vi "ComputeFourierPhaseOfPeakSF.vi"(6 "Header":T1, 9 "Search SF Limit":i32=20, 10 "FFT size":i32=256, 11 "Scan Frame":dbl[][](array[numeric])) -> (0 "Col Shift Element Number":i32, 1 "Vertical SF Phase":dbl, 2 "Row Shift Element Numbert":i32, 3 "Horizontal SF Phase":dbl)   [LabVIEW 2014]
uses:
  <vilib>/Analysis/baseanly.llb/Mean (DBL).vi
  <vilib>/Analysis/2dsp.llb/Real FFT.vi
  <vilib>/Analysis/NI_AALPro.lvlib
  <vilib>/Analysis/NI_AALBase.lvlib
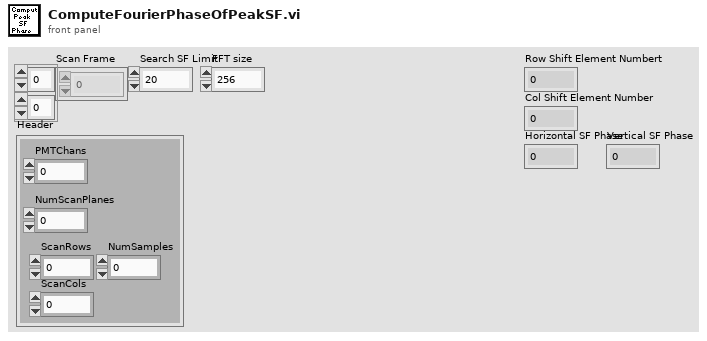
[diagram p1: front panel]
types:
  T1 = cluster{"PMTChans":i32, "NumScanPlanes":i32, "ScanRows":i32, "ScanCols":i32, "NumSamples":i32}
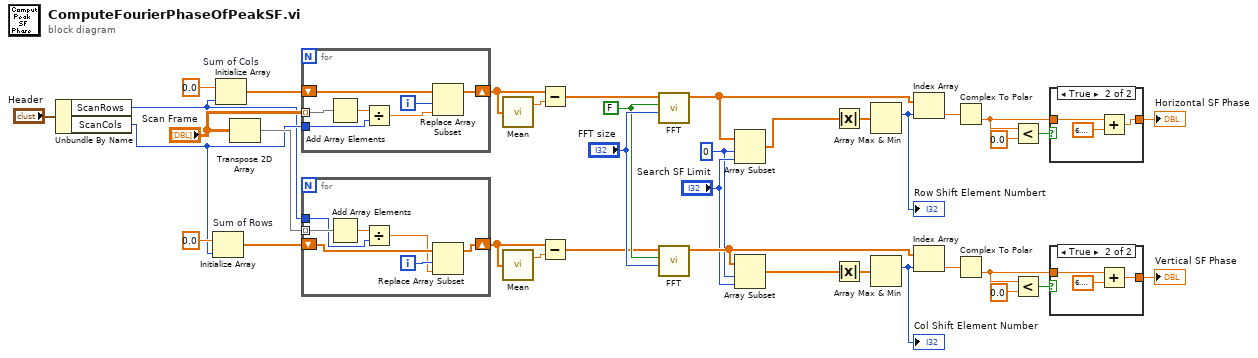
[diagram p0: block diagram]
diagram:
  w1 = 0 ("index")
  w29 = FALSE ("shift?")
  n1 = Unbundle By Name("Header") -> ("ScanRows"=w2:i32, "ScanCols"=w3:i32)
  n2 = Initialize Array "Sum of Rows"(0.0 ("element"), w3) -> (w33:dbl[])
  n3 = Initialize Array "Sum of Cols"(0.0 ("element"), w2) -> (w35:dbl[])
  n4 = Transpose 2D Array(2D array="Scan Frame") -> (transposed array=w34:dbl[][])
  n5 = for {
    tunnel: "Scan Frame" -> [w44] mode=indexing
    shift-right: [w42] -> w19
    shift-left: w35 -> [w43]
    tunnel: w3 -> [w39]
    i -> [w41]
    n6 = Add Array Elements(numeric array=w44) -> (sum=w40:dbl)
    n7 = Divide(x=w40, y=w39) -> (x/y=w38:dbl)
    n8 = Replace Array Subset(array=w43, new element=w38, index=w41) -> (w42:dbl[])
  }
  n9 = for {
    tunnel: w34 -> [w51] mode=indexing
    shift-right: [w49] -> w17
    shift-left: w33 -> [w50]
    tunnel: w2 -> [w46]
    i -> [w48]
    n10 = Add Array Elements(numeric array=w51) -> (sum=w47:dbl)
    n11 = Divide(x=w47, y=w46) -> (x/y=w45:dbl)
    n12 = Replace Array Subset(array=w50, new element=w45, index=w48) -> (w49:dbl[])
  }
  n13 = call-poly <vilib>:"Mean.vi"("X"=w19) -> ("mean"=w21:dbl)  [unwired: 1 out]
  n14 = call-poly <vilib>:"Mean.vi"("X"=w17) -> ("mean"=w18:dbl)  [unwired: 1 out]
  n15 = Subtract(x=w19, y=w21) -> (x-y=w20:dbl[])
  n16 = Subtract(x=w17, y=w18) -> (x-y=w16:dbl[])
  n17 = call-poly <vilib>:"FFT.vi"("FFT size"="FFT size", "shift?"=w29, "X"=w20) -> ("FFT {X}"=w23:cdb[])  [unwired: 7 in, 1 out]
  n18 = call-poly <vilib>:"FFT.vi"("FFT size"="FFT size", "shift?"=w29, "X"=w16) -> ("FFT {X}"=w22:cdb[])  [unwired: 7 in, 1 out]
  n19 = Array Subset(array=w23, index=w1, length="Search SF Limit") -> (w28:cdb[])
  n20 = Array Subset(array=w22, index=w1, length="Search SF Limit") -> (w26:cdb[])
  n21 = Absolute Value(x=w28) -> (abs(x)=w27:dbl[])
  n22 = Absolute Value(x=w26) -> (abs(x)=w25:dbl[])
  n23 = Array Max & Min(array=w27) -> (max index (indices)=w24:i32)  [unwired: 3 out]
  "Row Shift Element Numbert" <- w24
  n24 = Array Max & Min(array=w25) -> (max index (indices)=w14:i32)  [unwired: 3 out]
  "Col Shift Element Number" <- w14
  n25 = Index Array(array=w23, index=w24) -> (element=w13:cdb)
  n26 = Index Array(array=w22, index=w14) -> (element=w12:cdb)
  n27 = Complex To Polar(r * e^(i*theta)=w13) -> (theta=w9:dbl)  [unwired: 1 out]
  n28 = Complex To Polar(r * e^(i*theta)=w12) -> (theta=w6:dbl)  [unwired: 1 out]
  n29 = Less?(x=w9, y=0.0) -> (x < y?=w10:bool)
  n30 = Less?(x=w6, y=0.0) -> (x < y?=w7:bool)
  n31 = case shown="True" w10 {
    tunnel: w9 -> [w52 w55]
    tunnel: [w52 w53] -> w5
    frame False {
    }
    frame True {
      n32 = Add(x=w55, y=6.283185307179586) -> (x+y=w53:dbl)
    }
  }
  "Horizontal SF Phase" <- w5
  n33 = case shown="True" w7 {
    tunnel: w6 -> [w56 w59]
    tunnel: [w56 w57] -> w4
    frame False {
    }
    frame True {
      n34 = Add(x=w59, y=6.283185307179586) -> (x+y=w57:dbl)
    }
  }
  "Vertical SF Phase" <- w4
